vi "Calibration Control Loop.vi"   [LabVIEW 2014]
uses:
  <vilib>/Rock Robotics/Network Tables/SD Read Boolean.vi
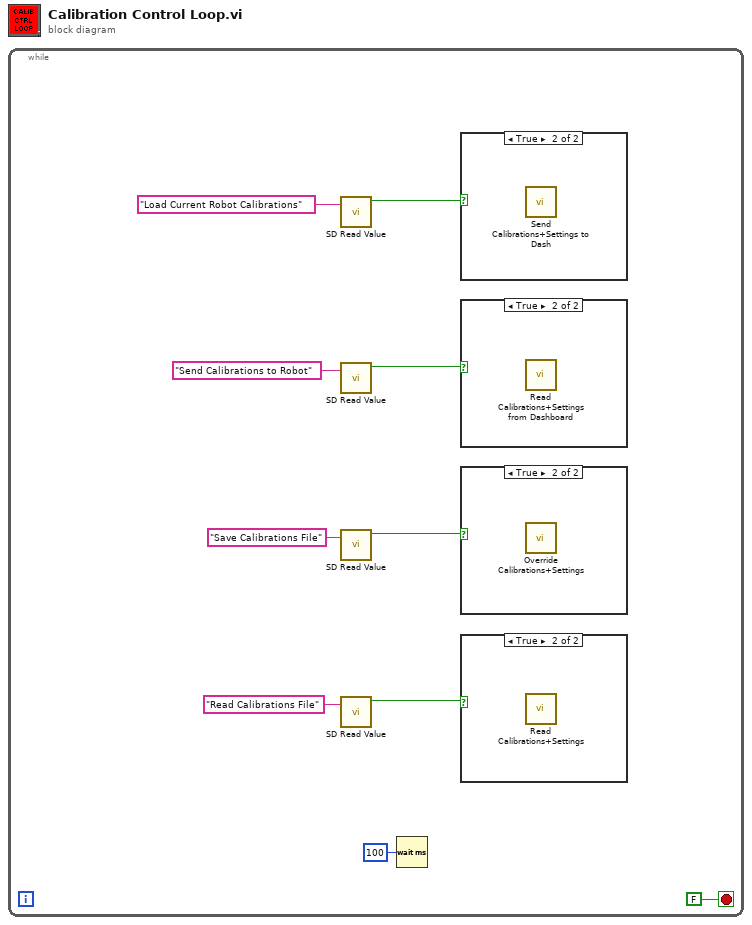
[diagram p0: block diagram]
diagram:
  n1 = while {
    stop <- FALSE stop-if-true
    n2 = call-poly <vilib>:"SD Read Value.vi"("Name"="Load Current Robot Calibrations") -> ("Boolean"=w6:bool)  [unwired: 8 in, 2 out]
    n3 = call-poly <vilib>:"SD Read Value.vi"("Name"="Send Calibrations to Robot") -> ("Boolean"=w3:bool)  [unwired: 8 in, 2 out]
    n4 = call-poly <vilib>:"SD Read Value.vi"("Name"="Save Calibrations File") -> ("Boolean"=w4:bool)  [unwired: 8 in, 2 out]
    n5 = call-poly <vilib>:"SD Read Value.vi"("Name"="Read Calibrations File") -> ("Boolean"=w5:bool)  [unwired: 8 in, 2 out]
    n6 = Wait (ms)(milliseconds to wait=u32 100) -> ()  [unwired: 1 out]
    n7 = case shown="True" w6 {
      frame False {
      }
      frame True {
        n8 = call "Send Calibrations+Settings to Dash.vi"() -> ()  [unwired: 12 in]
      }
    }
    n9 = case shown="True" w3 {
      frame False {
      }
      frame True {
        n10 = call "Read Calibrations+Settings from Dashboard.vi"() -> ()  [unwired: 12 in]
      }
    }
    n11 = case shown="True" w4 {
      frame False {
      }
      frame True {
        n12 = call "Override Calibrations+Settings.vi"() -> ()  [unwired: 12 in]
      }
    }
    n13 = case shown="True" w5 {
      frame False {
      }
      frame True {
        n14 = call "Read Calibrations+Settings.vi"() -> ()  [unwired: 12 in]
      }
    }
  }
